vi "Read Multiple.vi"(8 "error in":errorcluster, 11 "task in":i32) -> (0 "error out":errorcluster, 2 "data":u8[](array[numeric]), 3 "task out":i32)   [LabVIEW 2023, in "DO_Relay.lvlib"]
uses:
  <userlib>/DAQNavi Polymorphic VI/read/DAQNavi Read (Digital 1D U8 NChan 1Samp).vi
  DO_Relay.lvlib
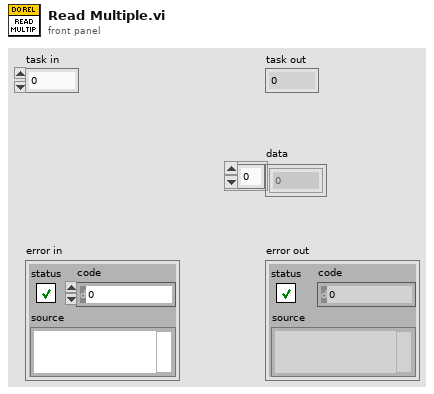
[diagram p1: front panel]
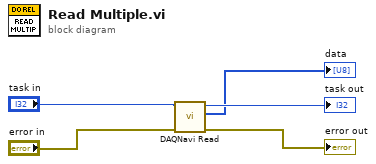
[diagram p0: block diagram]
diagram:
  n1 = call-poly <userlib>:"DAQNavi Read.vi"("error in (no error)"="error in", "task in"="task in") -> ("error out"=→"error out":errorcluster, "data"=→"data":u8[], "task out"=→"task out":i32)  [unwired: 1 in, 6 out]
